vi "Open Serial.vi"(8 "Error In":errorcluster, 10 "Baud Rate Override":u32, 11 "Serial Port":refnum<visa-resource-name>="N/A") -> (0 "Error Out":errorcluster={"status"=FALSE, "code"=1073676294, "source"="VISA Read in LVH-LINX.lvlib:Device.lvlib:Serial Read.vi->LVH-LINX.lvlib:Device.lvlib:Wait For Packet.vi->LVH-LINX.lvlib:Device.lvlib:Send Command.vi->LVH-LINX.lvlib:Device.lvlib:Get DIO Channels.vi->LVH-LINX.lvlib:Device.lvlib:Load Device Config.vi->LVH-LINX.lvlib:Device.lvlib:Initialize Device.vi->LVH-LINX.lvlib:Initialize.vi->Untitled 2"}, 2 "Device Name":string, 3 "LINX Resource":T1={"IO"=enum."Remote", "LINX Device Config"={"Interface"=enum."Serial", "COM Port"="COM13", "TCP Configuration"={"IP Address"="", "Port"=0}, "Device Family"=1, "Device ID"=1, "Device Name"="myRIO-1900", "TCP Ref"=refnum, "Local Refnum"=0, "Channels"={"DI"=[0, 1, 2, 3, 4, 5, 6, 7, 8, 9, 10, 11, 12, 13, 14, 15, 16, 17, 18, 19, 20, 21, 22, 23, 24, 25, 26, 27, 28, 29, 30, 31, 32, 33, 34, 35, 36, 37, 38, 39, 40, 41, 42, 43, 44, 45, 46], "DO"=[0, 1, 2, 3, 4, 5, 6, 7, 8, 9, 10, 11, 12, 13, 14, 15, 16, 17, 18, 19, 20, 21, 22, 23, 24, 25, 26, 27, 28, 29, 30, 31, 32, 33, 34, 35, 36, 37, 38, 39, 40, 41, 42, 43, 44, 45, 46], "AI"=[0, 1, 2, 3, 4, 5, 6, 7, 8, 9, 10, 11], "AO"=[], "PWM"=[3, 5, 6, 9, 10], "QE"=[], "UART"=[0, 1], "I2C 2"=[0], "SPI"=[0], "CAN"=[], "Servo"=[], "AI Ref (V)"=0.0, "AI Resolution (Bits)"=0, "AO Ref (V)"=0.0, "AO Resolution (Bits)"=0}}})   [LabVIEW 2020, in "LMH-LINX.lvlib"]
doc: "Open a serial connection to a remote LINX device."
uses:
  LMH-LINX.lvlib
  Private/Type Defs/LINX Ref.ctl
  Private/Type Defs/Platform.ctl
  Private/Device/Type Defs/LINX Device Config.ctl
  Private/Type Defs/Interface.ctl
  Private/Device/Type Defs/TCP Config.ctl
  Private/Device/Type Defs/Channels.ctl
  Private/Type Defs/User Platform.ctl
  Private/Device/Device.lvlib
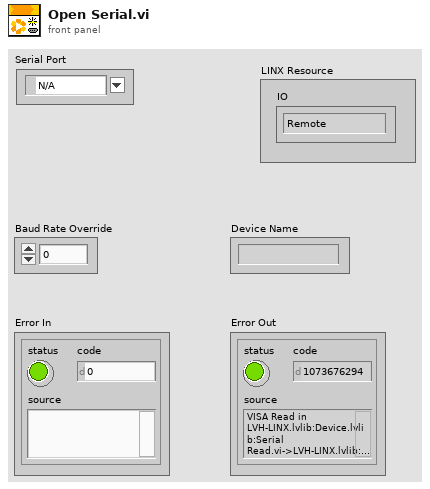
[diagram p1: front panel]
types:
  T1 = typedef "LMH-LINX.lvlib/LINX Ref.ctl" = cluster{"IO":T2, "LINX Device Config":T3}
  T2 = typedef "LMH-LINX.lvlib/Platform.ctl" = enum16{"Remote", "Local"}
  T3 = typedef "Device.lvlib/LINX Device Config.ctl" = cluster{"Interface":T4, "COM Port":refnum<visa-resource-name>, "TCP Configuration":T5, "Device Family":u8, "Device ID":u8, "Device Name":string, "TCP Ref":refnum<k5>, "Local Refnum":u64, "Channels":T6}
  T4 = typedef "LMH-LINX.lvlib/Interface.ctl" = enum16{"Serial", "TCP"}
  T5 = typedef "Device.lvlib/TCP Config.ctl" = cluster{"IP Address":string, "Port":u16}
  T6 = typedef "LMH-LINX.lvlib/Channels.ctl" = cluster{"DI":u8[], "DO":u8[], "AI":u8[], "AO":u8[], "PWM":u8[], "QE":u8[], "UART":u8[], "I2C 2":u8[], "SPI":u8[], "CAN":u8[], "Servo":u8[], "AI Ref (V)":dbl, "AI Resolution (Bits)":u8, "AO Ref (V)":dbl, "AO Resolution (Bits)":u8}
  T7 = typedef "LMH-LINX.lvlib/User Platform.ctl" = enum16{"Default", "Remote", "Local"}
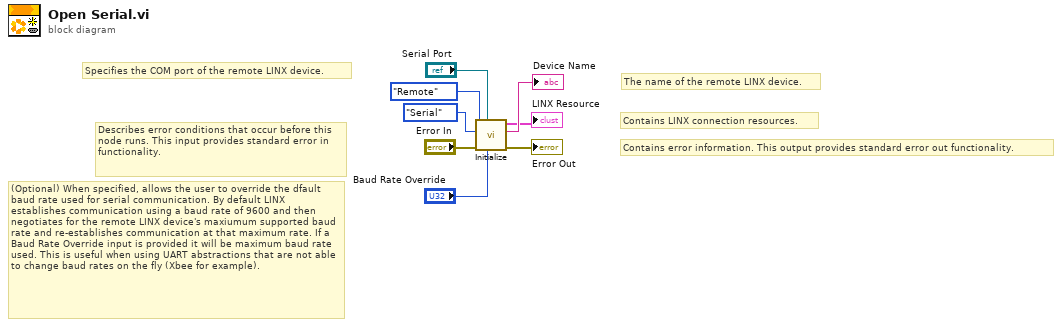
[diagram p0: block diagram]
diagram:
  # "Contains error information. This output provides standard error out functionality."
  # "Contains LINX connection resources."
  # "The name of the remote LINX device."
  # "(Optional) When specified, allows the user to override the dfault baud rate used for serial communication. By default LINX establishes communication using a baud rate of 9600 and then negotiates for the remote LINX device's maxiumum supported baud rate and re-establishes communication at that maximum rate. If a Baud Rate Override input is provided it will be maximum baud rate used. This is useful when using UART abstractions that are not able to change baud rates on the fly (Xbee for example)."
  # "Describes error conditions that occur before this node runs. This input provides standard error in functionality."
  # "Specifies the COM port of the remote LINX device."
  n1 = call "Initialize.vi"("Baud Rate Override"="Baud Rate Override", "Serial Port"="Serial Port", "Error In"="Error In", "Interface"=Interface."Serial", "IO"=User_Platform."Remote" ("Platform")) -> ("Error Out"=→"Error Out":errorcluster, "Device Name"=→"Device Name":string, "LINX Resource"=→"LINX Resource":T1)  [unwired: 4 in]
